vi "keysight_read.vi"(0 "error in":errorcluster, 2 "command":string, 3 "Connection":T1={"Type"=1, "VISA"="TCPIP0::192.168.0.8::inst0::INSTR", "GPIB"="10"} {"Type" items=["VISA", "GPIB"]}) -> (1 "error out":errorcluster={"status"=TRUE, "code"=-1073807343, "source"="VISA Open in keysight_read.vi"}, 4 "Raw output":string)   [LabVIEW 2013]
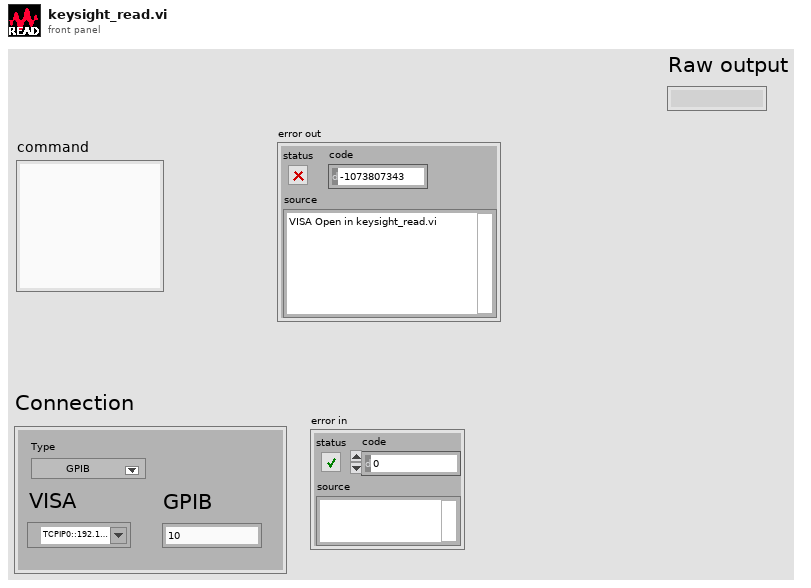
[diagram p1: front panel]
types:
  T1 = cluster{"Type":u16, "VISA":refnum<visa-resource-name>, "GPIB":string}
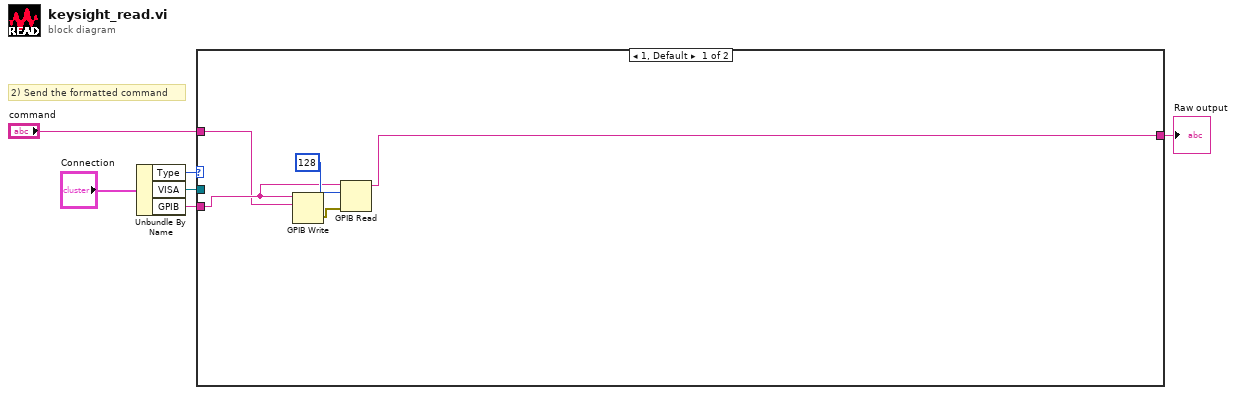
[diagram p0: block diagram]
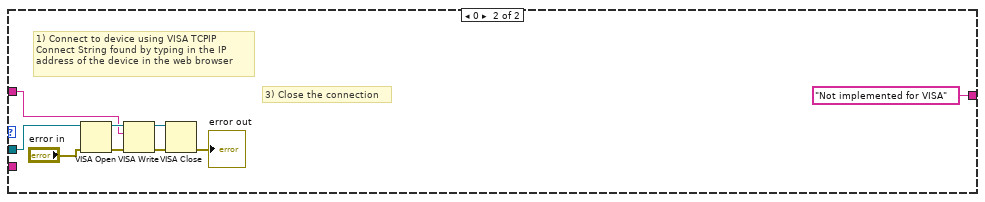
[diagram p2: hidden frame]
diagram:
  # "2) Send the formatted command"
  n1 = Unbundle By Name("Connection") -> ("Type"=w4:u16, "VISA"=w3:refnum<visa-resource-name>, "GPIB"=w2:string)
  n2 = case shown="1, Default" w4 {
    tunnel: "command" -> [w8 w15]
    tunnel: w2 -> [w9 _]
    tunnel: w3 -> [_ w13]
    tunnel: [w7 "Not implemented for VISA" ("data")] -> w1
    frame 1, Default {
      n3 = GPIB Write(0:w9, 1:w8) -> (6:w11:errorcluster)  [unwired: 3 in, 1 out]
      n4 = GPIB Read(0:w9, 1:128, 3:w11) -> (5:w7:string)  [unwired: 2 in, 2 out]
    }
    frame 0 {
      # "3) Close the connection"
      # "1) Connect to device using VISA TCPIP Connect String found by typing in the IP address of the device in the web browser"
      n5 = VISA Open(error in (no error)="error in", VISA resource name=w13) -> (VISA resource name=w16:refnum<visa-resource-name>, error out=w17:errorcluster)  [unwired: 3 in]
      n6 = VISA Write(VISA resource name=w16, write buffer=w15, error in (no error)=w17) -> (VISA resource name out=w18:refnum<visa-resource-name>, error out=w19:errorcluster)  [unwired: 1 out]
      n7 = VISA Close(VISA resource name=w18, error in (no error)=w19) -> (error out=→"error out":errorcluster)
    }
  }
  "Raw output" <- w1
